vi "Handle Mouse Up.vi"(8 "error in (no error)":errorcluster, 9 "Mouse Coordinates":T1, 11 "Toolbar Control in":refnum<class "Toolbar Control.lvclass">) -> (0 "error out":errorcluster, 1 "Button Name":string, 2 "Button State":T2, 3 "Toolbar Control out":refnum<class "Toolbar Control.lvclass">, 5 "Icon Index Over":i32)   [LabVIEW 2011, in "Toolbar Control.lvclass"]
doc: "This VI handles the Mouse Up event on the toolbar. When the Mouse Up event is detected run this VI providing the current <B>Mouse Coordinates</B>. This VI will then return the information about the icon that the mouse is over. But this does not mean the user has made their selection, they may have clicked the More Options item which shows more items to choose from.\n\n-------------\nDeveloped by Brian Hoover (hooovahh)"
uses:
  Toolbar Control.lvclass
  Controls/Button State.ctl
  <vilib>/Utility/miscctls.llb/LVPoint32TypeDef.ctl
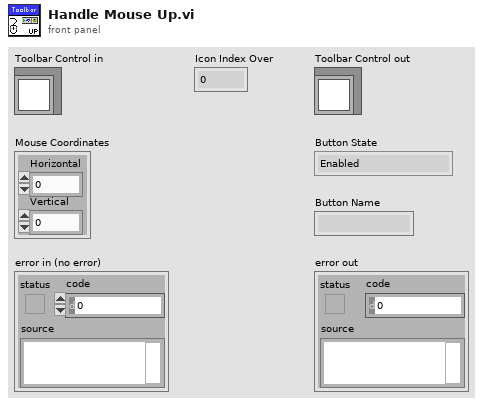
[diagram p1: front panel]
types:
  T1 = typedef "LVPoint32TypeDef.ctl" = cluster{"Horizontal":i32, "Vertical":i32}
  T2 = typedef "Toolbar Control.lvclass/Button State.ctl" = enum8{"Enabled", "Disabled", "Disabled and Grayed Out"}
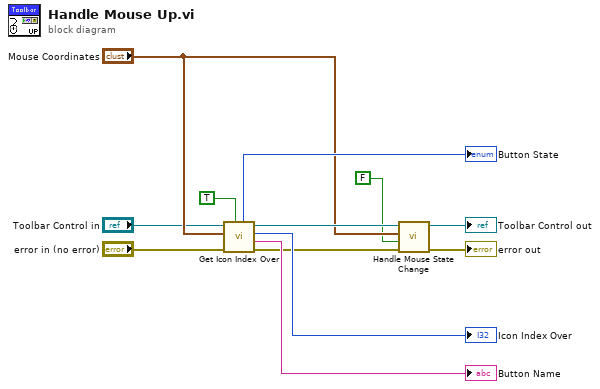
[diagram p0: block diagram]
diagram:
  n1 = call "Get Icon Index Over.vi"("UI Mouse Up"=TRUE, "error in (no error)"="error in (no error)", "Mouse Coordinates"="Mouse Coordinates", "Toolbar Control in"="Toolbar Control in") -> ("error out"=w8:errorcluster, "Button Name"=→"Button Name":string, "Icon Index Over"=→"Icon Index Over":i32, "Toolbar Control out"=w7:refnum<class "Toolbar Control.lvclass">, "Button State"=→"Button State":T2)  [unwired: 3 in]
  n2 = call "Handle Mouse State Change.vi"("error in (no error)"=w8, "Mouse Down"=FALSE ("Boolean"), "Mouse Coordinates"="Mouse Coordinates", "Toolbar Control in"=w7) -> ("error out"=→"error out":errorcluster, "Toolbar Control out"=→"Toolbar Control out":refnum<class "Toolbar Control.lvclass">)  [unwired: 4 in, 2 out]
